vi "Fit Transform.vi"(8 "error in (no error)":errorcluster caption="entrée d'erreur (pas d'erreur)", 10 "y":string[][](array[string]), 11 "LabelEncoder.lvclass":refnum<class "LabelEncoder.lvclass">) -> (0 "error out":errorcluster caption="sortie d'erreur", 2 "Data":T1, 3 "LabelEncoder.lvclass":refnum<class "LabelEncoder.lvclass">)   [LabVIEW 2020, in "LabelEncoder.lvclass"]
doc: "Fit label encoder and return encoded labels\n\nReturns : \n\n- y : array-like of shape [n_samples]"
uses:
  LabelEncoder.lvclass
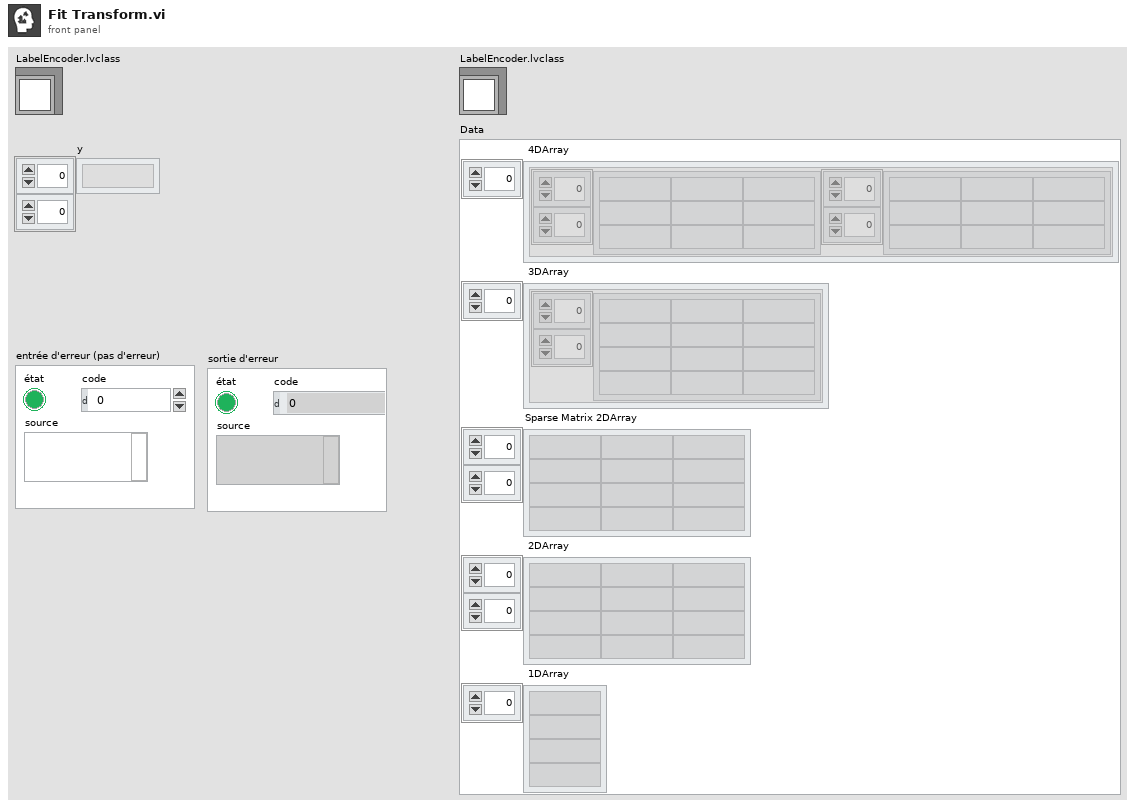
[diagram p1: front panel]
types:
  T1 = cluster{" 4DArray":cluster{"1":string[][], "2":string[][]}[], " 3DArray":cluster{"Tableau":string[][]}[], "Sparse Matrix 2DArray":string[][], " 2DArray":string[][], " 1DArray":string[]}
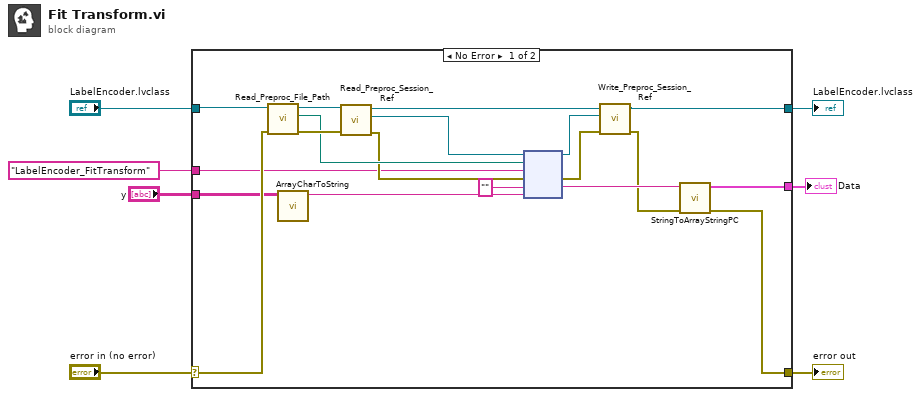
[diagram p0: block diagram]
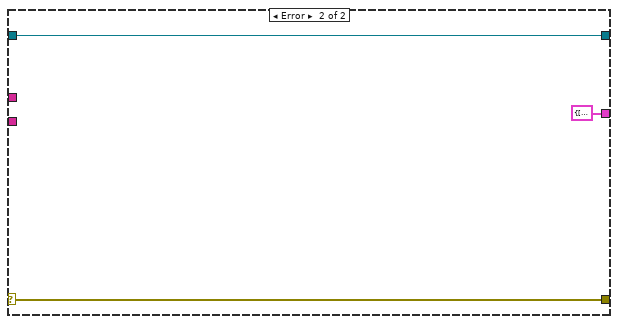
[diagram p2: hidden frame]
diagram:
  n1 = case shown="No Error" "error in (no error)" {
    selector: "error in (no error)" -> [w17 w29]
    tunnel: [w8 w29] -> w6
    tunnel: [w10 w28] -> w4
    tunnel: "LabelEncoder.lvclass" -> [w16 w28]
    tunnel: "LabelEncoder_FitTransform" ("Fonction") -> [w15 _]
    tunnel: [w9 T1 {" 4DArray"=[], " 3DArray"=[], "Sparse Matrix 2DArray"=[], " 2DArray"=[], " 1DArray"=[]} ("Data")] -> w2
    tunnel: "y" -> [w14 _]
    frame No Error {
      n2 = call-dynamic "Read_Preproc_File_Path.vi"("error in (no error)"=w17, "Python in"=w16) -> ("error out"=w25:errorcluster, "File_Path"=w22:path, "Python out"=w26:refnum<class "LabelEncoder.lvclass">)  [unwired: 7 in]
      n3 = call "ArrayCharToString.vi"("TAB"=w14) -> ("Instruction"=w13:string)  [unwired: 10 in]
      n4 = call-dynamic "Read_Preproc_Session_Ref.vi"("error in (no error)"=w25, "Python in"=w26) -> ("error out"=w21:errorcluster, "Session_ref"=w23:refnum<k35>, "Python out"=w24:refnum<class "LabelEncoder.lvclass">)  [unwired: 7 in]
      n5 = node(w23, w22, w15, w21, "", w13) -> (w19:refnum<k35>, w20:errorcluster, w12:string)  [unwired: 1 in, 2 out]
      n6 = call-dynamic "Write_Preproc_Session_Ref.vi"("error in (no error)"=w20, "Session_ref"=w19, "Python in"=w24) -> ("error out"=w11:errorcluster, "Python out"=w10:refnum<class "LabelEncoder.lvclass">)  [unwired: 7 in]
      n7 = call "StringToArrayStringPC.vi"("sortie d'erreur"=w11, "Return value"=w12) -> ("sortie d'erreur"=w8:errorcluster, "Data"=w9:T1)  [unwired: 8 in]
    }
    frame Error {
    }
  }
  "error out" <- w6
  "LabelEncoder.lvclass" <- w4
  "Data" <- w2
